vi "SwitchedDMM.vi"(4 "DMM Class":string="Sim DMM\\Sim DMM.lvclass", 5 "Setting":T1={"Resolution (Digits)"=5.5, "Current Source (Amps)"=0.001, "Range"=2.0, "Measurement Type"=enum."4-wire Resistance"} {"Resolution (Digits)" items=["3 1/2"=3.5, "4 1/2"=4.5, "5 1/2"=5.5, "6 1/2"=6.5, "7 1/2"=7.5]; "Current Source (Amps)" items=["1uA"=1e-06, "10uA"=1e-05, "100uA"=0.0001, "1mA"=0.001]}, 6 "DMM Resource":string, 7 "Connection(s)":string="ch49->com3", 8 "error in":errorcluster, 9 "Switch Resource":string, 10 "Switch Class":string="Sim Switch\\Sim Switch.lvclass", 11 "Base Path":path=path "C:/GitHub/OOP Template/HAL/Concrete") -> (0 "error out":errorcluster={"status"=TRUE, "code"=1059, "source"="Get LV Class Default Value.vi<APPEND>\n\n<b>Complete call chain:</b>\r\n     Get LV Class Default Value.vi\r\n     MAL.lvlib:SwitchedDMM.vi\r\n\r\n<b>LabVIEW attempted to load the class at this path:</b>\r\nC:\\GitHub\\OOP Template\\HAL\\Concrete\\Sim Switch"}, 3 "Measurements":dbl)   [LabVIEW 2019, in "MAL.lvlib"]
uses:
  MAL.lvlib
  Hardware Abstraction/Harware Abstraction/Switch/Switch.lvclass
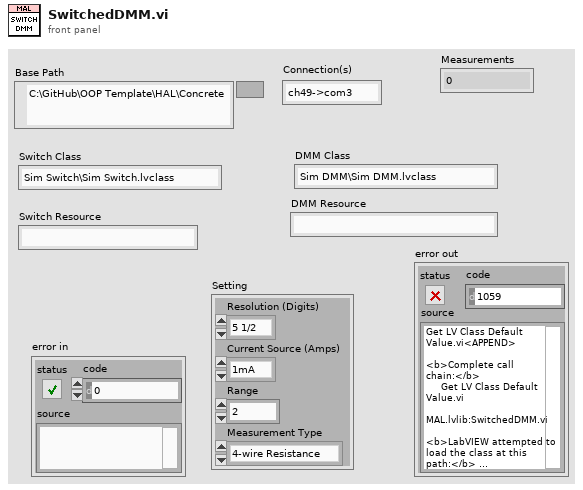
[diagram p1: front panel]
types:
  T1 = cluster{"Resolution (Digits)":dbl, "Current Source (Amps)":dbl, "Range":dbl, "Measurement Type":enum16{"DC Volts", "AC Volts", "DC Current", "AC Current", "2-wire Resistance", "4-wire Resistance", "Diode", "Frequency", "Period", "AC Volts DC Coupled", "Capacitance", "Inductance", "Temperature"}}
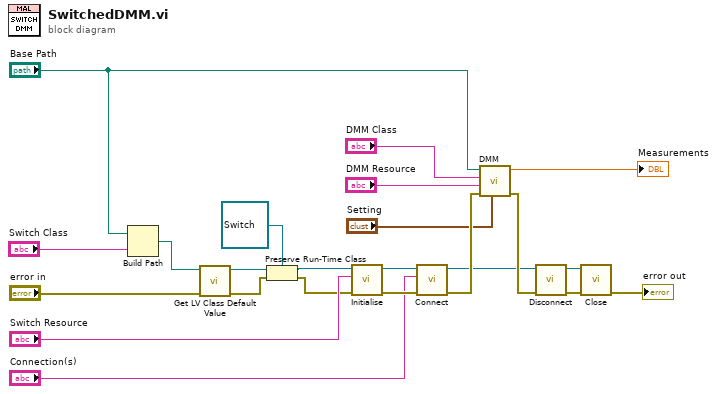
[diagram p0: block diagram]
diagram:
  n1 = Build Path(base path="Base Path", name or relative path="Switch Class") -> (appended path=w3:path)
  n2 = call <vilib>:"Get LV Class Default Value.vi"("error in (no error)"="error in", "class path"=w3) -> ("error out"=w21:errorcluster, "object"=w22:refnum<class>)  [unwired: 8 in]
  n3 = Preserve Run-Time Class(object in=w22, error in=w21, 2:refnum<class "Switch.lvclass"> refnum ("Hardware Abstration.lvlib:Switch.lvclass")) -> (object out=w19:refnum<class "Switch.lvclass">, error out=w18:errorcluster)
  n4 = call-dynamic "Initialise.vi"("error in (no error)"=w18, "Instrument Ref"="Switch Resource", "Instrument in"=w19) -> ("error out"=w16:errorcluster, "Instrument out"=w15:refnum<class "Switch.lvclass">)  [unwired: 7 in]
  n5 = call-dynamic "Connect.vi"("error in (no error)"=w16, "Channel(s)"="Connection(s)", "Switch in"=w15) -> ("error out"=w11:errorcluster, "Switch out"=w9:refnum<class "Switch.lvclass">)  [unwired: 7 in]
  n6 = call "DMM.vi"("Setting"="Setting", "error in"=w11, "DMM Ref"="DMM Resource", "DMM Class"="DMM Class", "Base Path"="Base Path") -> ("error out"=w10:errorcluster, "Measurements"=→"Measurements":dbl)  [unwired: 5 in]
  n7 = call-dynamic "Disconnect.vi"("error in (no error)"=w10, "Switch in"=w9) -> ("error out"=w14:errorcluster, "Switch out"=w13:refnum<class "Switch.lvclass">)  [unwired: 8 in]
  n8 = call-dynamic "Close.vi"("error in (no error)"=w14, "Instrument in"=w13) -> ("error out"=→"error out":errorcluster)  [unwired: 8 in, 1 out]
